vi "RSZVB Set Generator Frequency Conversion.vi"(0 "VISA session":refnum<visa-resource-name>, 1 "Channel (1)":i32=1, 2 "Port (1)":i32=1, 3 "Generator Number (1)":i32=1, 4 "State (F: Off)":bool, 5 "error in (no error)":errorcluster {"code" format="%.0x"}, 6 "Denominator (1)":i32=1, 7 "Offset (0.0)":dbl format="%^.3e", 8 "Sweep Type (0: Sweep)":i32(ring) items=["Sweep", "CW/Fixed"], 9 "Numerator (1)":i32=1) -> (14 "dup VISA session":refnum<visa-resource-name>, 19 "error out":errorcluster {"code" format="%.0x"})   [LabVIEW 2011]
doc: "This VI defines an external generator frequency for frequency-converting measurements. The external generator frequency is either a range (for frequency sweeps) or a CW frequency (for power, time and CW Mode sweeps).\n\nNote(s):\n\n(1) This VI is available only on R&S ZVA instrument.\n\nRemote-control command(s):\nSOURce<Ch>:FREQuency<Pt>:CONVersion:ARBitrary:EFRequency<Gen> \n<Boolean>, <numerator>, <denominator>, <offset>, CW | FIXed | SWEep"
uses:
  _utility/RSZVB Global Data.vi
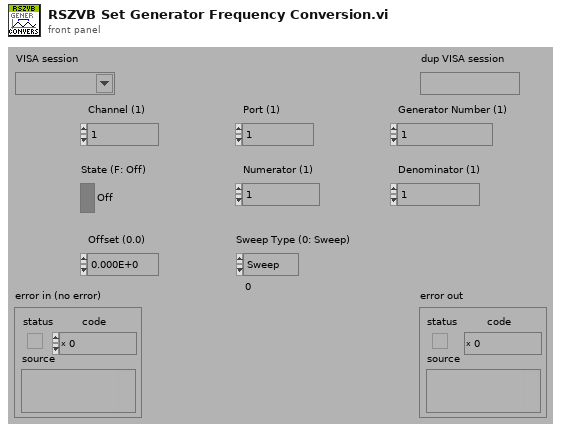
[diagram p1: front panel]
types:
  T1 = cluster{"Error Checking (T: On)":bool, "Installed Options":string[], "Data Valid?":bool, "Ports":i32, "Model":string[], "Option Checking (T: On)":bool}[]
  T2 = cluster{"Error Checking (T: On)":bool, "Installed Options":string[], "Data Valid?":bool, "Ports":i32, "Model":string[], "Option Checking (T: On)":bool}
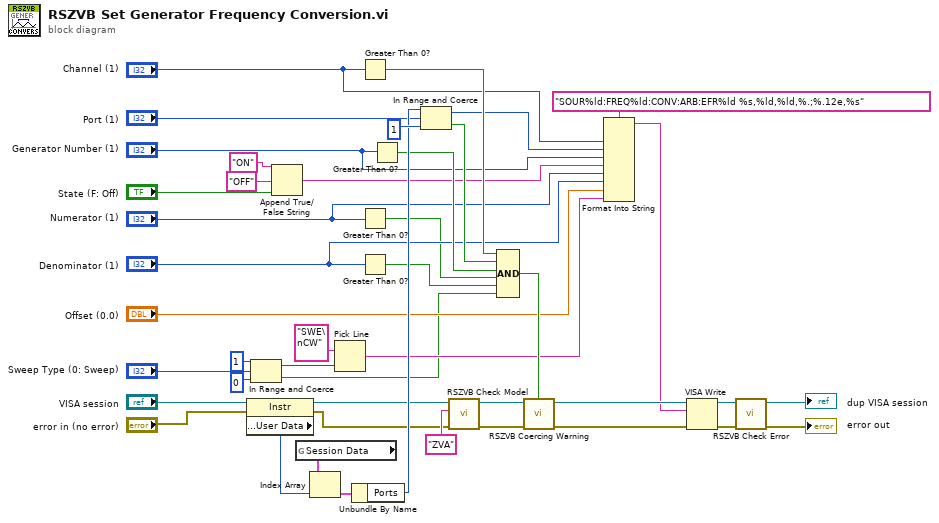
[diagram p0: block diagram]
diagram:
  n1 = property class="Instr"(reference="VISA session", error in="error in (no error)") -> (reference out=w26:refnum<visa-resource-name>, error out=w25:errorcluster, "General Settings:User Data"=w43:u32)
  n2 = In Range and Coerce(upper limit=1 ("lower limit"), x="Sweep Type (0: Sweep)", lower limit=0) -> (coerced(x)=w31:i32, In Range?=w1:bool)
  n3 = Append True/False String(1:"State (F: Off)", 2:"OFF", 3:"ON") -> (0:w8:string)  [unwired: 1 in]
  n4 = global read "RSZVB Global Data.vi" "Session Data"() -> (w42:T1)
  n5 = Index Array(array=w42, index=w43) -> (element=w41:T2)
  n6 = Pick Line(multi-line string="SWE\nCW", line index=w31) -> (output string=w5:string)  [unwired: 1 in]
  n7 = Unbundle By Name(w41) -> ("Ports"=w35:i32)
  n8 = Greater Than 0?(x="Channel (1)") -> (x > 0?=w40:bool)
  n9 = Greater Than 0?(x="Numerator (1)") -> (x > 0?=w4:bool)
  n10 = Greater Than 0?(x="Denominator (1)") -> (x > 0?=w3:bool)
  n11 = Greater Than 0?(x="Generator Number (1)") -> (x > 0?=w10:bool)
  n12 = In Range and Coerce(upper limit=w35, x="Port (1)", lower limit=1) -> (coerced(x)=w18:i32, In Range?=w14:bool)
  n13 = call "RSZVB Check Model.vi"("error in (no error)"=w25, "Model"="ZVA" ("Options"), "VISA session"=w26) -> ("error out"=w28:errorcluster, "dup VISA session"=w27:refnum<visa-resource-name>)  [unwired: 7 in]
  n14 = Compound Arithmetic op=AND(w40, w14, w10, w4, w3, w1) -> (w39:bool)
  n15 = call "RSZVB Coercing Warning.vi"("In Range?"=w39, "error in (no error)"=w28, "VISA session"=w27) -> ("error out"=w30:errorcluster, "dup VISA session"=w36:refnum<visa-resource-name>)  [unwired: 7 in]
  n16 = Format Into String(format string="SOUR%ld:FREQ%ld:CONV:ARB:EFR%ld %s,%ld,%ld,%.;%.12e,%s", "Channel (1)", w18, "Generator Number (1)", w8, "Numerator (1)", "Denominator (1)", "Offset (0.0)", w5) -> (resulting string=w15:string)  [unwired: 2 in, 1 out]
  n17 = VISA Write(VISA resource name=w36, write buffer=w15, error in (no error)=w30) -> (VISA resource name out=w38:refnum<visa-resource-name>, error out=w37:errorcluster)  [unwired: 1 out]
  n18 = call "RSZVB Check Error.vi"("error in (no error)"=w37, "VISA session"=w38) -> ("error out"=→"error out":errorcluster, "dup VISA session"=→"dup VISA session":refnum<visa-resource-name>)  [unwired: 8 in]
